vi "demo.vi"() -> ()   [LabVIEW 2023]
uses:
  C:/Users/tommaso/Desktop/touchDiverCS_DLL/touchDiverCS4_DLL/bin/Debug/touchDiverCS4_DLL.dll
  touchDiverCS4_DLL/bin/Debug/touchDiverCS4_DLL.dll
panel:
  in  "ttValue":i32
  out "number":dbl
  out "String":string
  in  "Combo Box":string(combo)
  in  "Force":sgl(slide) min=0 max=1 step=0.05 scale=0.0..1.0
  in  "Temperature":sgl(slide) min=0 max=1 step=0.05 scale=0.0..1.0
  in  "stop":bool
  in  "start Haptics":bool
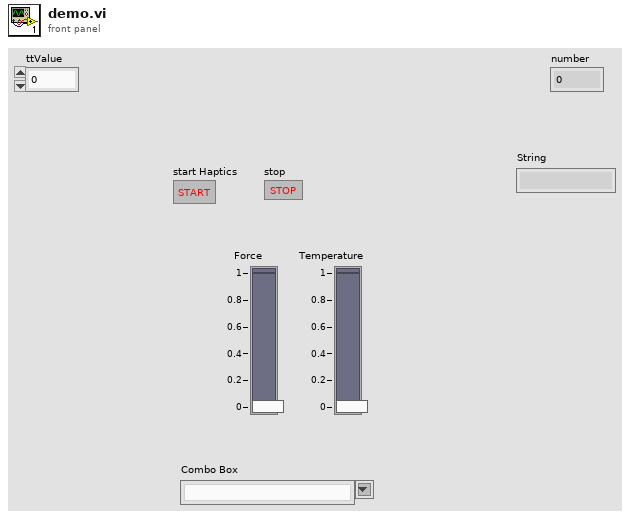
[diagram p1: front panel]
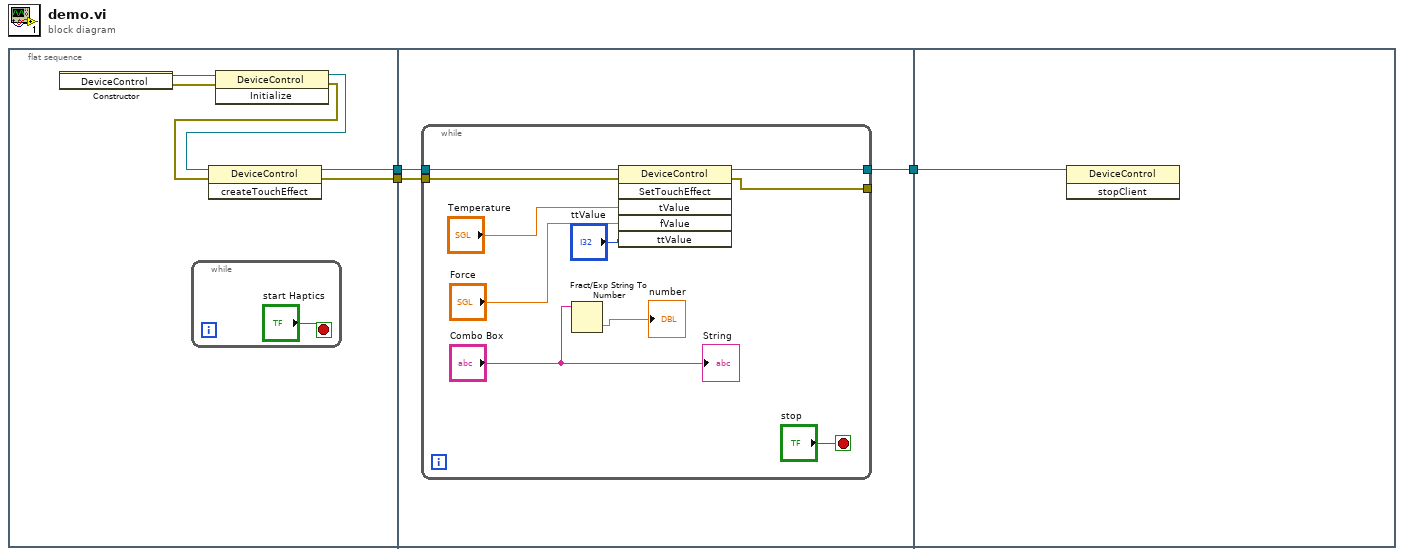
[diagram p0: block diagram]
diagram:
  n1 = flat-sequence {
    tunnel: [w8] -> w3
    tunnel: [w6] -> w1
    tunnel: w3 -> [w13]
    tunnel: [w12] -> w2
    tunnel: w1 -> [w11]
    tunnel: w2 -> [w24]
    frame #0 {
      n2 = constructor class="DeviceControl"() -> (reference out=w5:refnum<k24>, error out=w4:errorcluster)  [unwired: 3 in, 1 out]
      n3 = while {
        stop <- "start Haptics" stop-if-true
      }
      n4 = invoke class="DeviceControl" method="Initialize"(reference=w5, error in=w4) -> (reference out=w9:refnum<k24>, error out=w7:errorcluster)  [unwired: 1 in, 1 out]
      n5 = invoke class="DeviceControl" method="createTouchEffect"(reference=w9, error in=w7) -> (reference out=w8:refnum<k24>, error out=w6:errorcluster)  [unwired: 1 in, 1 out]
    }
    frame #1 {
      n6 = while {
        tunnel: w13 -> [w22]
        tunnel: [w19] -> w12
        tunnel: w11 -> [w18]
        tunnel: [w17] -> _
        stop <- "stop" stop-if-true
        n7 = Fract/Exp String To Number(string="Combo Box") -> (number=→"number":dbl)  [unwired: 3 in, 1 out]
        n8 = invoke class="DeviceControl" method="SetTouchEffect"(reference=w22, error in=w18, "tValue"="Temperature", "fValue"="Force", "ttValue"="ttValue") -> (reference out=w19:refnum<k24>, error out=w17:errorcluster)  [unwired: 1 in, 4 out]
        "String" <- "Combo Box"
      }
    }
    frame #2 {
      n9 = invoke class="DeviceControl" method="stopClient"(reference=w24) -> ()  [unwired: 2 in, 3 out]
    }
  }
